vi "output.vi"(8 "error in":errorcluster, 10 "output data table":T1, 11 "shared memory module":refnum<class "Shared Memory Runtime.lvclass">) -> (0 "error out":errorcluster, 2 "output data table out":T1, 3 "shared memory module out":refnum<class "Shared Memory Runtime.lvclass">)   [LabVIEW 2013, in "Shared Memory Runtime.lvclass"]
doc: "Provides an interface for information processing by a module at runtime. While this interface performs no operations, a child should provide an override which may process data in any manner necessary.Copyright 2016 National Instruments Corporation\n\nLicensed under the Apache License, Version 2.0 (the \"License\"); you may not use this file except in compliance with the License. You may obtain a copy of the License at http://www.apache.org/licenses/LICENSE-2.0\nUnless required by applicable law or agreed to in writing, software distributed under the License is distributed on an \"AS IS\" BASIS, WITHOUT WARRANTIES OR CONDITIONS OF ANY KIND, either express or implied. See the License for the specific language governing permissions and limitations under the License."
uses:
  Shared Memory Runtime.lvclass
  <vilib>/NI/Tag Bus/table/data table.ctl
  Shared Memory Runtime.lvclass/Shared Memory Runtime.ctl
  <vilib>/NI/Tag Bus/table/data polymorphs/read many/read Doubles.vi
  <vilib>/NI/Tag Bus/table/data table.lvlib
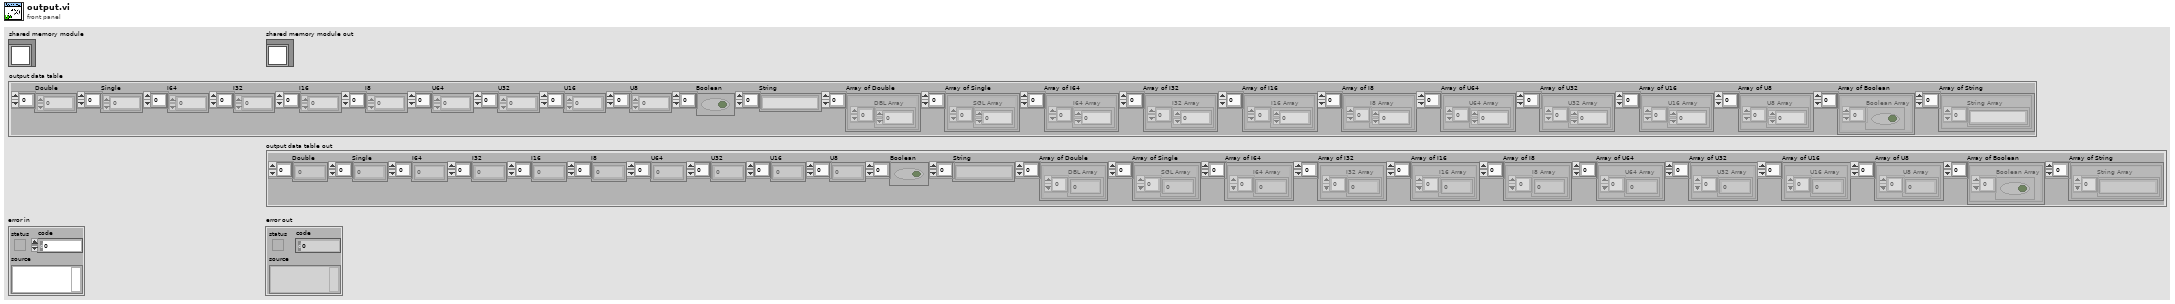
[diagram p1: front panel]
types:
  T1 = typedef "tag bus.lvlib/data table.lvlib/data table.ctl" = cluster{"Double":dbl[], "Single":sgl[], "I64":i64[], "I32":i32[], "I16":i16[], "I8":i8[], "U64":u64[], "U32":u32[], "U16":u16[], "U8":u8[], "Boolean":bool[], "String":string[], "Array of Double":cluster{"DBL Array":dbl[]}[], "Array of Single":cluster{"SGL Array":sgl[]}[], "Array of I64":cluster{"I64 Array":i64[]}[], "Array of I32":cluster{"I32 Array":i32[]}[], "Array of I16":cluster{"I16 Array":i16[]}[], "Array of I8":cluster{"I8 Array":i8[]}[], "Array of U64":cluster{"U64 Array":u64[]}[], "Array of U32":cluster{"U32 Array":u32[]}[], "Array of U16":cluster{"U16 Array":u16[]}[], "Array of U8":cluster{"U8 Array":u8[]}[], "Array of Boolean":cluster{"Boolean Array":bool[]}[], "Array of String":cluster{"String Array":string[]}[]}
  T2 = typedef "Shared Memory Runtime.lvclass/shared memory module runtime.ctl" = cluster{"refnum":refnum<file>, "name":string, "data type":T3, "number of tags":i32, "indices":cluster{"index":i32[]}, "data array":cluster{"data":dbl[]}, "file array":cluster{"data":dbl[]}}
  T3 = typedef "tag bus.lvlib/tag descriptor.lvclass/Data Type.ctl" = enum16{"Double", "Single", "I64", "I32", "I16", "I8", "U64", "U32", "U16", "U8", "Boolean", "String", "Array of Double", "Array of Single", "Array of I64", "Array of I32", "Array of I16", "Array of I8", "Array of U64", "Array of U32", "Array of U16", "Array of U8", "Array of Boolean", "Array of String"}
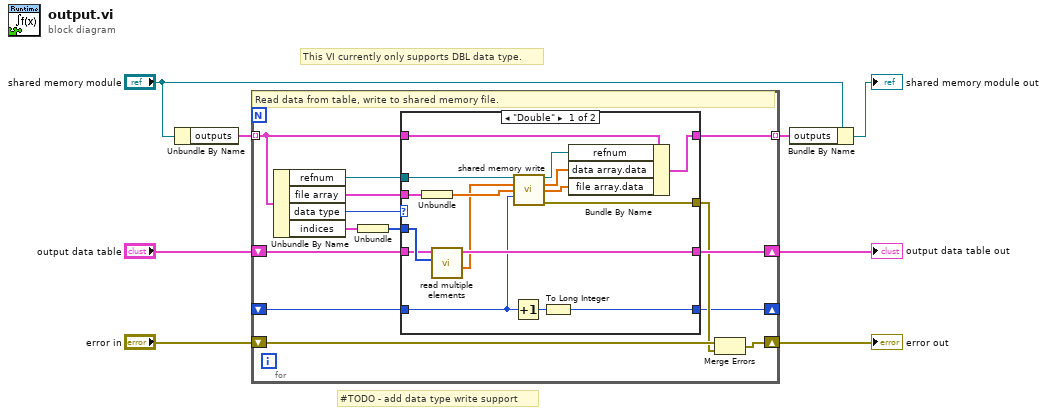
[diagram p0: block diagram]
diagram:
  # "#TODO - add data type write support"
  # "This VI currently only supports DBL data type."
  n1 = Unbundle By Name("shared memory module") -> ("outputs"=w8:T2[])
  n2 = for {
    tunnel: w8 -> [w10] mode=indexing
    shift-right: [w21] -> w6
    shift-left: "error in" -> [w22]
    shift-right: [w17] -> w4
    shift-left: "output data table" -> [w20]
    shift-right: [w11] -> _
    shift-left: _ -> [w12]
    tunnel: [w9] -> w2 mode=indexing
    # "Read data from table, write to shared memory file."
    n3 = Unbundle By Name(w10) -> ("refnum"=w13:refnum<file>, "file array"=w15:cluster{"data":dbl[]}, "data type"=w18:T3, "indices"=w19:cluster{"index":i32[]})
    n4 = Unbundle(w19) -> ("index"=w16:i32[])
    n5 = case shown="\"Double\"" w18 {
      tunnel: w16 -> [w38 _]
      tunnel: w20 -> [w37 w41]
      tunnel: [w36 w41] -> w17
      tunnel: w15 -> [w35 _]
      tunnel: [w28 _] -> w14
      tunnel: w13 -> [w34 _]
      tunnel: w12 -> [w31 w40]
      tunnel: [w29 w40] -> w11
      tunnel: w10 -> [w27 w39]
      tunnel: [w23 w39] -> w9
      frame "Double" {
        n6 = Unbundle(w35) -> ("data"=w33:dbl[])
        n7 = call-poly <vilib>:"read multiple elements.vi"("indices"=w38, "data table in"=w37) -> ("values"=w32:dbl[], "data table out"=w36:T1)  [unwired: 8 in]
        n8 = Increment(x=w31) -> (x+1=w30:i32)
        n9 = call "shared memory write.vi"("refnum in"=w34, "Data Array"=w32, "File Array Allocation"=w33, "Counter"=w31) -> ("refnum out"=w26:refnum<file>, "Data Array Out"=w25:dbl[], "File Array Allocation Out"=w24:dbl[], "error out"=w28:errorcluster)  [unwired: 8 in]
        n10 = To Long Integer(number=w30) -> (32bit integer=w29:i32)
        n11 = Bundle By Name(cluster=w27, "refnum"=w26, "data array.data"=w25, "file array.data"=w24) -> (w23:T2)
      }
      frame Default {
      }
    }
    n12 = Merge Errors(w22, w14) -> (w21:errorcluster)
  }
  "error out" <- w6
  "output data table out" <- w4
  n13 = Bundle By Name(cluster="shared memory module", "outputs"=w2) -> (→"shared memory module out":refnum<class "Shared Memory Runtime.lvclass">)
